vi "Shooting.vi"(6 "Shoot override":dbl, 7 "Serializer Override":dbl, 9 "Lock PWM":bool) -> (0 "Serializer Output":dbl=0.5, 1 "Feeder Output":dbl=1.0, 2 "Shooter PWM":dbl=0.7440168132715996, 3 "Rotation Out":dbl=0.09822222222222224)   [LabVIEW 2016]
uses:
  <vilib>/Rock Robotics/Network Tables/NT Read Number.vi
  <vilib>/Rock Robotics/Network Tables/NT Read Numeric Array.vi
  Robot Global Data.vi
  <vilib>/addons/control/pid/pid.llb/PID (DBL).vi
  <vilib>/addons/control/pid/NI_PID_pid.lvlib
panel:
  in  "Disable PID?":bool=TRUE
  out "Image width":dbl(graph)
  out "Object Width":dbl=21.666666666666668
  out "Ball In?":i16(graph)
  out "PWM Output":dbl(graph)
  in  "Lower limit 2":dbl=-3.1 format="%#_13g"
  in  "upper limit 2":dbl=3.1 format="%#_13g"
  out "Object X direct output":dbl(graph)=-7.888888888888889
  out "Offset":dbl=5.0 format="%#_13g"
  in  "Lower limit":dbl=-0.1 format="%#_13g"
  in  "upper limit":dbl=0.1 format="%#_13g"
  in  "PID gains":T1={"proportional gain (Kc)"=0.052, "integral time (Ti, min)"=0.0, "derivative time (Td, min)"=0.002} {"derivative time (Td, min)" format="%.3f"; "integral time (Ti, min)" format="%.3f"; "proportional gain (Kc)" format="%.3f"}
  # "Does nothing, only used as a template for the incoming values from DB"
  # "Practice Bot\nP: 0.052\nI: 0\nD: 0.002"
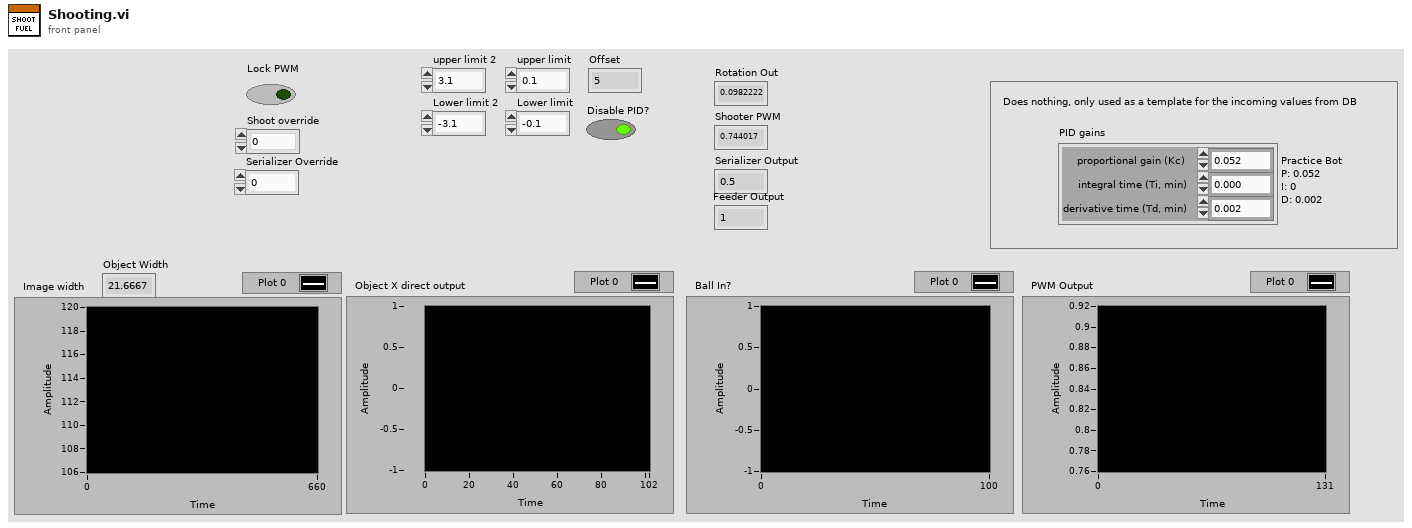
[diagram p1: front panel]
types:
  T1 = cluster{"proportional gain (Kc)":dbl, "integral time (Ti, min)":dbl, "derivative time (Td, min)":dbl}
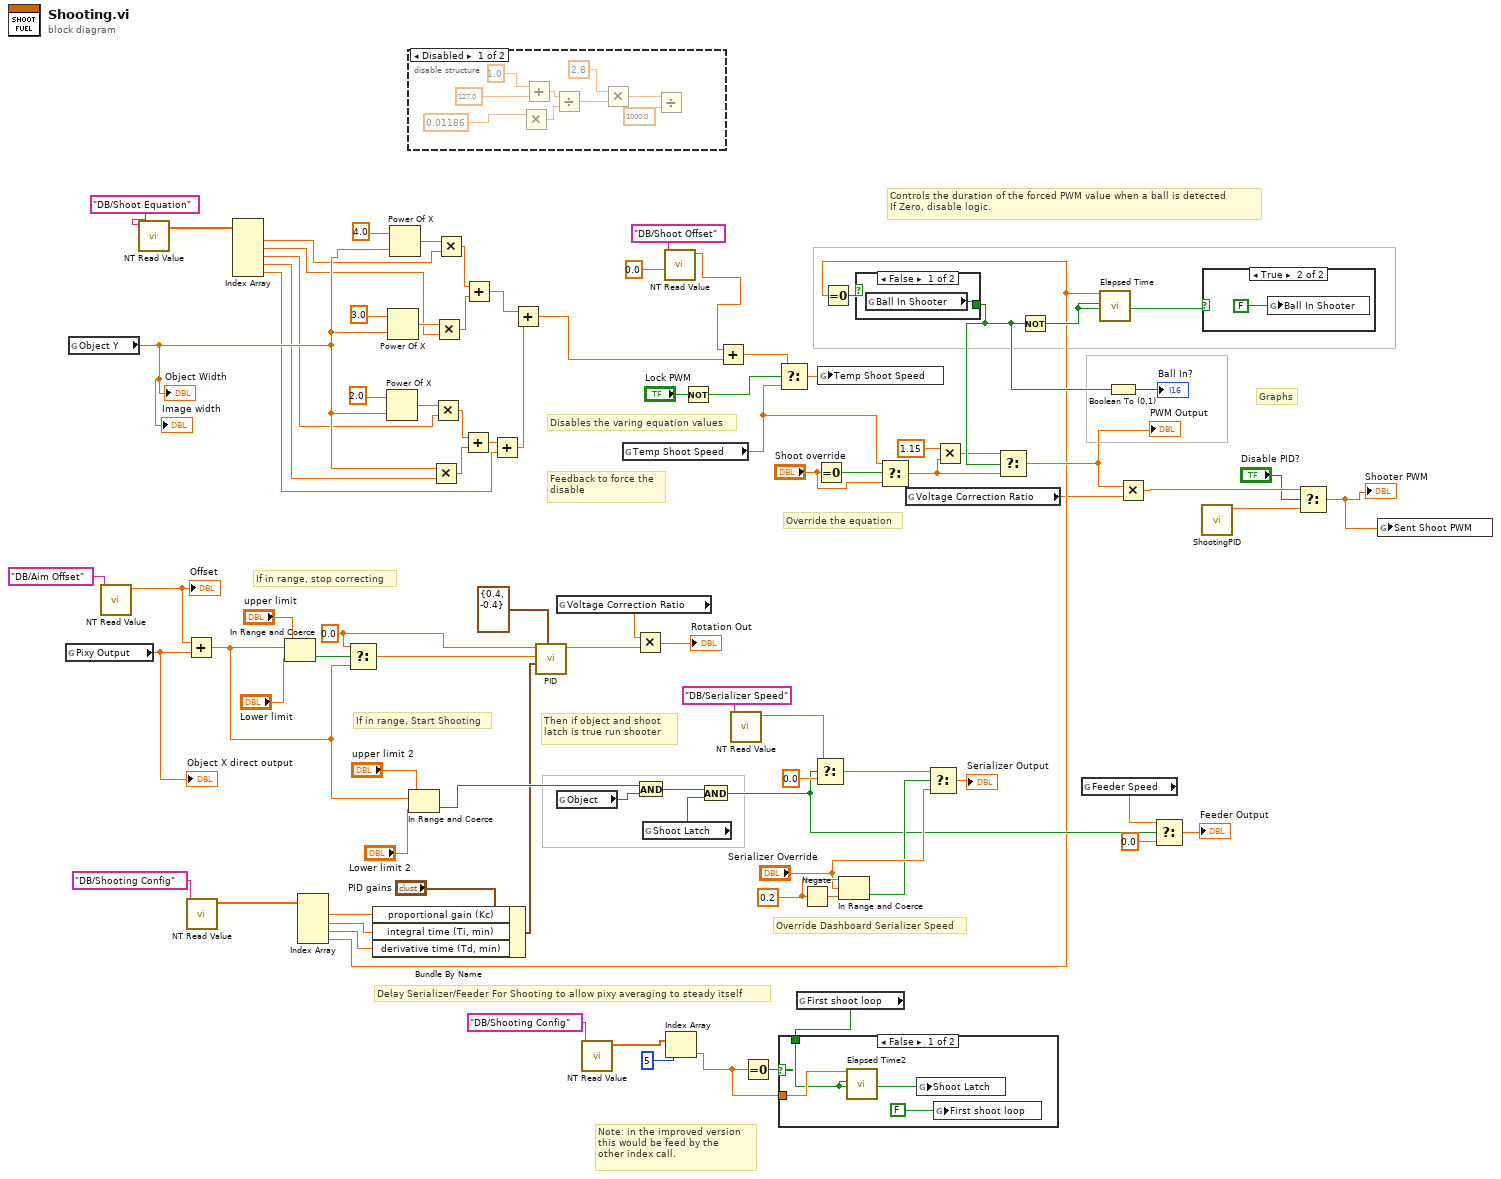
[diagram p0: block diagram]
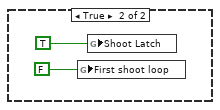
[diagram p2: hidden frame]
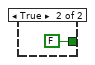
[diagram p3: hidden frame]
diagram:
  w78 = 0.0
  w87 = 0.2
  # "Note: in the improved version\nthis would be feed by the\nother index call."
  # "Then if object and shoot \nlatch is true run shooter"
  # "If in range, Start Shooting"
  # "If in range, stop correcting"
  # "Controls the duration of the forced PWM value when a ball is detected\nIf Zero, disable logic."
  # "Graphs"
  # "Feedback to force the\ndisable"
  # "Disables the varing equation values"
  # "Override the equation"
  # "Delay Serializer/Feeder For Shooting to allow pixy averaging to steady itself"
  # "Override Dashboard Serializer Speed"
  n1 = global read "Robot Global Data.vi" "Pixy Output"() -> (w76:dbl)
  "Object X direct output" <- w76
  n2 = global read "Robot Global Data.vi" "Object Y"() -> (w13:dbl)
  "Object Width" <- w13
  "Image width" <- w13
  n3 = call-poly <vilib>:"NT Read Value.vi"("Name"="DB/Aim Offset") -> ("Numeric"=w59:dbl)  [unwired: 9 in, 1 out]
  "Offset" <- w59
  n4 = call-poly <vilib>:"NT Read Value.vi"("Name"="DB/Shoot Equation") -> ("Numeric Array"=w11:dbl[])  [unwired: 9 in, 1 out]
  n5 = Add(x=w59, y=w76) -> (x+y=w72:dbl)
  n6 = call-poly <vilib>:"NT Read Value.vi"("Name"="DB/Shooting Config") -> ("Numeric Array"=w57:dbl[])  [unwired: 9 in, 1 out]
  n7 = Index Array(array=w11) -> (element #1=w10:dbl, element #2=w9:dbl, element #3=w8:dbl, element #4=w7:dbl, element #5=w6:dbl)  [unwired: 5 in]
  n8 = In Range and Coerce(upper limit="upper limit", x=w72, lower limit="Lower limit") -> (In Range?=w73:bool)  [unwired: 1 out]
  n9 = Index Array(array=w57) -> (element #1=w55:dbl, element #2=w54:dbl, element #3=w53:dbl, element #4=w36:dbl)  [unwired: 4 in]
  n10 = Select(t=w78, s=w73, f=w72) -> (s? t:f=w80:dbl)
  n11 = Bundle By Name(cluster="PID gains", "proportional gain (Kc)"=w55, "integral time (Ti, min)"=w54, "derivative time (Td, min)"=w53) -> (w52:T1)
  n12 = Power Of X(1:w13, 2:2.0 ("x")) -> (0:w21:dbl)
  n13 = Power Of X(1:w13, 2:3.0 ("x")) -> (0:w23:dbl)
  n14 = Power Of X(1:w13, 2:4.0 ("x")) -> (0:w25:dbl)
  n15 = disable-structure shown="Disabled" {
    frame Disabled {
      n16 = Multiply(x=0.01186) -> (x*y=w96:dbl)  [unwired: 1 in]
      n17 = Add(x=1.0, y=127.0) -> (x+y=w100:dbl)
      n18 = Divide(x=w100, y=w96) -> (x/y=w99:dbl)
      n19 = Multiply(x=2.8, y=w99) -> (x*y=w93:dbl)
      n20 = Divide(x=w93, y=1000.0) -> ()  [unwired: 1 out]
    }
    frame Enabled {
    }
  }
  n21 = In Range and Coerce(upper limit="upper limit 2", x=w72, lower limit="Lower limit 2") -> (In Range?=w71:bool)  [unwired: 1 out]
  n22 = Multiply(x=w13, y=w7) -> (x*y=w17:dbl)
  n23 = Multiply(x=w21, y=w8) -> (x*y=w18:dbl)
  n24 = Multiply(x=w23, y=w9) -> (x*y=w19:dbl)
  n25 = Multiply(x=w25, y=w10) -> (x*y=w20:dbl)
  n26 = Add(x=w18, y=w17) -> (x+y=w16:dbl)
  n27 = Add(x=w20, y=w19) -> (x+y=w14:dbl)
  n28 = Add(x=w16, y=w6) -> (x+y=w15:dbl)
  n29 = Add(x=w14, y=w15) -> (x+y=w5:dbl)
  n30 = call-poly <vilib>:"PID.vi"("output range"=cluster{"output high":dbl, "output low":dbl} {"output high"=0.4, "output low"=-0.4}, "PID gains"=w52, "process variable"=w80, "setpoint"=w78) -> ("output"=w84:dbl)  [unwired: 6 in, 1 out]
  n31 = global read "Robot Global Data.vi" "Voltage Correction Ratio"() -> (w27:dbl)
  n32 = global read "Robot Global Data.vi" "Object"() -> (w68:bool)
  n33 = call-poly <vilib>:"NT Read Value.vi"("Name"="DB/Shooting Config") -> ("Numeric Array"=w33:dbl[])  [unwired: 9 in, 1 out]
  n34 = global read "Robot Global Data.vi" "Temp Shoot Speed"() -> (w62:dbl)
  n35 = Multiply(x=w27, y=w84) -> (x*y=→"Rotation Out":dbl)
  n36 = And(x=w71, y=w68) -> (x .and. y?=w48:bool)
  n37 = global read "Robot Global Data.vi" "Shoot Latch"() -> (w47:bool)
  n38 = call-poly <vilib>:"NT Read Value.vi"("Default Value"=0.0, "Name"="DB/Shoot Offset") -> ("Numeric"=w65:dbl)  [unwired: 8 in, 1 out]
  n39 = Index Array(array=w33, index=5) -> (element=w31:dbl)
  n40 = Not(x="Lock PWM") -> (.not. x?=w70:bool)
  n41 = And(x=w48, y=w47) -> (x .and. y?=w46:bool)
  n42 = Add(x=w65, y=w5) -> (x+y=w67:dbl)
  n43 = call-poly <vilib>:"NT Read Value.vi"("Name"="DB/Serializer Speed") -> ("Numeric"=w91:dbl)  [unwired: 9 in, 1 out]
  n44 = Equal To 0?(x=w31) -> (x = 0?=w35:bool)
  n45 = Select(t=w67, s=w70, f=w62) -> (s? t:f=w79:dbl)
  n46 = global read "Robot Global Data.vi" "First shoot loop"() -> (w30:bool)
  n47 = case shown="False" w35 {
    tunnel: w31 -> [w105 _]
    tunnel: w30 -> [w102 _]
    frame False {
      n48 = call "Elapsed Time2"("Time Target (s)"=w105, "Reset"=w102, "Auto Reset"=w102) -> ("Time has Elapsed"=w104:bool)  [unwired: 9 in, 7 out]
      n49 = global write "Robot Global Data.vi" "Shoot Latch"(w104) -> ()
      n50 = global write "Robot Global Data.vi" "First shoot loop"(FALSE ("Time has Elapsed")) -> ()
    }
    frame True {
      n51 = global write "Robot Global Data.vi" "First shoot loop"(FALSE ("Time has Elapsed")) -> ()
      n52 = global write "Robot Global Data.vi" "Shoot Latch"(TRUE ("Time has Elapsed")) -> ()
    }
  }
  n53 = Negate(x=w87) -> (-x=w88:dbl)
  n54 = Select(t=w91, s=w46, f=0.0) -> (s? t:f=w86:dbl)
  n55 = Equal To 0?(x="Shoot override") -> (x = 0?=w63:bool)
  n56 = global write "Robot Global Data.vi" "Temp Shoot Speed"(w79) -> ()
  n57 = Equal To 0?(x=w36) -> (x = 0?=w37:bool)
  n58 = In Range and Coerce(upper limit=w87, x="Serializer Override", lower limit=w88) -> (In Range?=w77:bool)  [unwired: 1 out]
  n59 = case shown="False" w37 {
    tunnel: [w108 FALSE ("Ball In Shooter")] -> w42
    frame False {
      n60 = global read "Robot Global Data.vi" "Ball In Shooter"() -> (w108:bool)
    }
    frame True {
    }
  }
  n61 = Select(t=w62, s=w63, f="Shoot override") -> (s? t:f=w38:dbl)
  n62 = global read "Robot Global Data.vi" "Voltage Correction Ratio"() -> (w29:dbl)
  n63 = Select(t=w86, s=w77, f="Serializer Override") -> (s? t:f=→"Serializer Output":dbl)
  n64 = Multiply(x=1.15 ("t"), y=w38) -> (x*y=w39:dbl)
  n65 = Select(t=w39, s=w42, f=w38) -> (s? t:f=w51:dbl)
  "PWM Output" <- w51
  n66 = Not(x=w42) -> (.not. x?=w49:bool)
  n67 = global read "Robot Global Data.vi" "Feeder Speed"() -> (w44:dbl)
  n68 = call "Elapsed Time"("Time Target (s)"=w36, "Reset"=w49, "Auto Reset"=w49) -> ("Time has Elapsed"=w50:bool)  [unwired: 9 in, 7 out]
  n69 = Boolean To (0,1)(Boolean=w42) -> (0, 1=→"Ball In?":i16)
  n70 = Multiply(x=w51, y=w29) -> (x*y=w4:dbl)
  n71 = Select(t=w44, s=w46, f=0.0) -> (s? t:f=→"Feeder Output":dbl)
  n72 = call "ShootingPID.vi"() -> ("Output"=w3:dbl)  [unwired: 11 in]
  n73 = case shown="True" w50 {
    frame False {
    }
    frame True {
      n74 = global write "Robot Global Data.vi" "Ball In Shooter"(FALSE) -> ()
    }
  }
  n75 = Select(t=w4, s="Disable PID?", f=w3) -> (s? t:f=w2:dbl)
  "Shooter PWM" <- w2
  n76 = global write "Robot Global Data.vi" "Sent Shoot PWM"(w2) -> ()
